vi "Read Length Y.vi"(8 "error in (no error)":errorcluster, 11 "ODESimulator_LinearConveyor in":refnum<class "ODESimulator_LinearConveyor.lvclass">) -> (0 "error out":errorcluster, 2 "Length Y":sgl=1.0, 3 "ODESimulator_LinearConveyor out":refnum<class "ODESimulator_LinearConveyor.lvclass">)   [LabVIEW 2017, in "NI_Robotics_Simulator.lvlib" / "ODESimulator_LinearConveyor.lvclass"]
uses:
  <vilib>/robotics/Simulator/Robot Factory/Conveyor/Linear/ODESimulator_LinearConveyor.lvclass
  <vilib>/robotics/Simulator/Robot Factory/Conveyor/Linear/ODESimulator_LinearConveyor.lvclass/ODESimulator_LinearConveyor.ctl
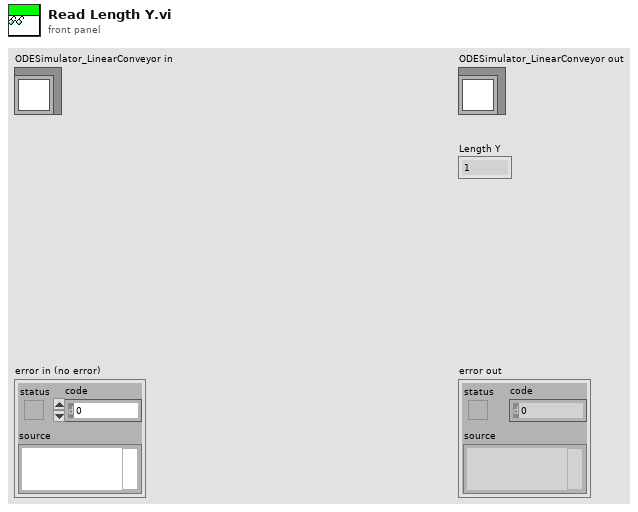
[diagram p1: front panel]
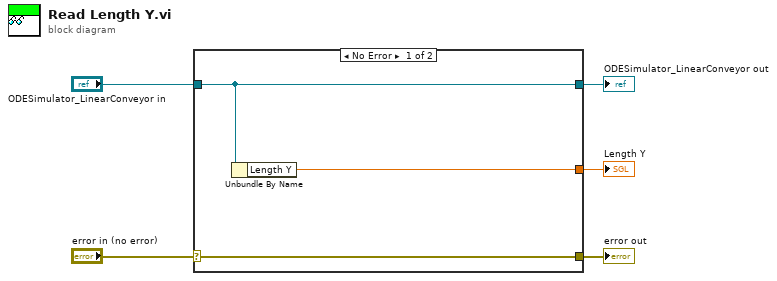
[diagram p0: block diagram]
diagram:
  n1 = case shown="No Error" "error in (no error)" {
    selector: "error in (no error)" -> [w8 w9]
    tunnel: [w8 w9] -> w4
    tunnel: [w7 w10] -> w2
    tunnel: "ODESimulator_LinearConveyor in" -> [w7 w10]
    tunnel: [w6 _] -> w1
    frame No Error {
      n2 = Unbundle By Name(w7) -> ("Length Y"=w6:sgl)
    }
    frame Error {
    }
  }
  "error out" <- w4
  "ODESimulator_LinearConveyor out" <- w2
  "Length Y" <- w1
